vi "TestListen.vi"(0 "Input cluster":T1, 1 "Test Ready":bool, 2 "Loop Number":i32, 5 "Max No. of Tests":i32=3, 7 "Time to Complete":dbl, 9 "% Complete":i32, 11 "No. of Test":i32=1, 12 "TF IN":bool) -> (3 "Test No.":i32, 4 "Queue cluster":T1, 6 "Test Param":T2, 8 "Voltage/(g/s)":bool, 13 "TF OUT":bool, 14 "State":i32)   [LabVIEW 2014]
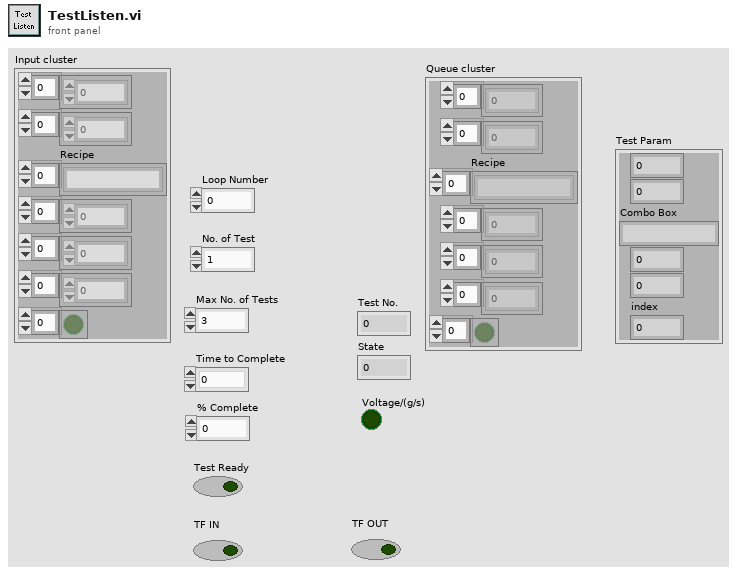
[diagram p1: front panel]
types:
  T1 = cluster{i32[], i32[], "Recipe":string[], i32[], i32[], i32[], bool[]}
  T2 = cluster{i32, i32, "Combo Box":string, i32, i32, "index":i32}
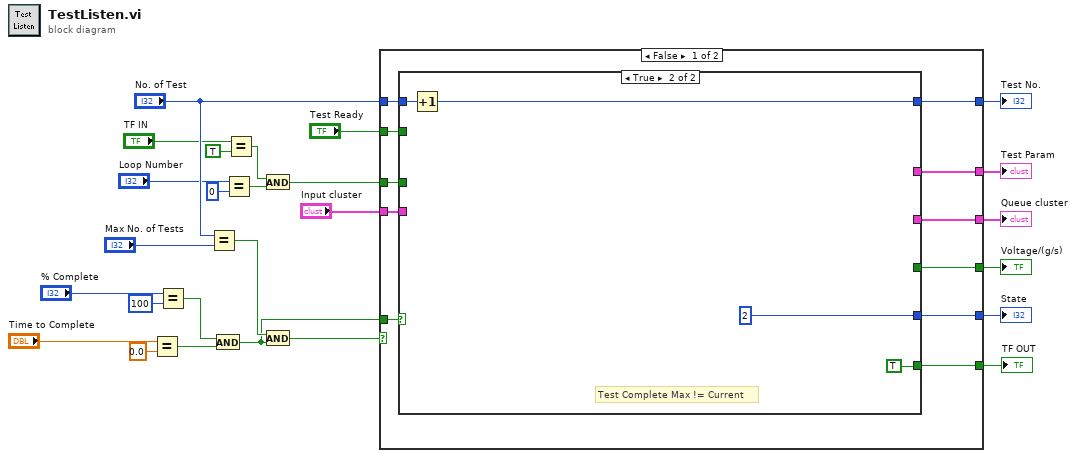
[diagram p0: block diagram]
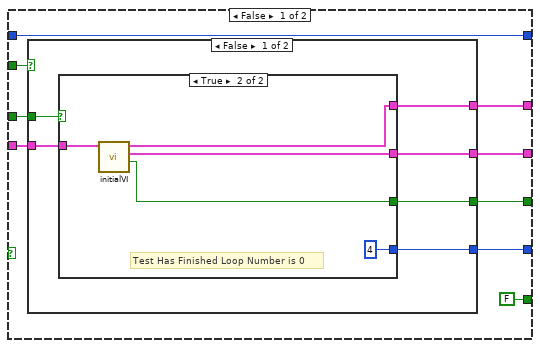
[diagram p2: hidden frame]
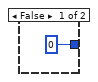
[diagram p3: hidden frame]
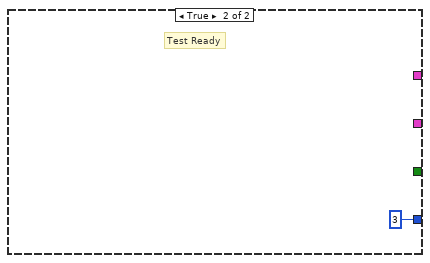
[diagram p4: hidden frame]
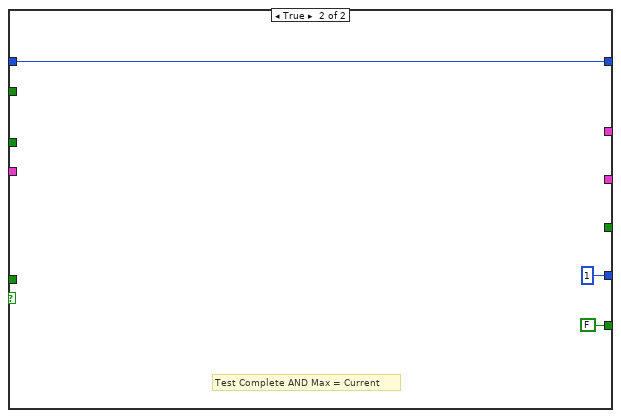
[diagram p5: hidden frame]
diagram:
  n1 = Equal?(x="Time to Complete", y=0.0) -> (x = y?=w24:bool)
  n2 = Equal?(x="% Complete", y=100) -> (x = y?=w25:bool)
  n3 = Equal?(x="No. of Test", y="Max No. of Tests") -> (x = y?=w26:bool)
  n4 = And(x=w25, y=w24) -> (x .and. y?=w21:bool)
  n5 = Equal?(x="Loop Number", y=0) -> (x = y?=w5:bool)
  n6 = Equal?(x="TF IN", y=TRUE) -> (x = y?=w3:bool)
  n7 = And(x=w3, y=w5) -> (x .and. y?=w2:bool)
  n8 = And(x=w26, y=w21) -> (x .and. y?=w22:bool)
  n9 = case shown="False" w22 {
    tunnel: w21 -> [w37 _]
    tunnel: "Test Ready" -> [w36 _]
    tunnel: [w35 1] -> w12
    tunnel: [w34 w65] -> w17
    tunnel: "No. of Test" -> [w33 w65]
    tunnel: w2 -> [w32 _]
    tunnel: "Input cluster" -> [w31 _]
    tunnel: [w30 _] -> w9
    tunnel: [w29 _] -> w11
    tunnel: [w28 _] -> w8
    tunnel: [w27 FALSE ("Test Ready 2")] -> w1
    frame False {
      n10 = case shown="True" w37 {
        tunnel: w36 -> [w45 _]
        tunnel: [w46 2] -> w35
        tunnel: [w44 w62] -> w34
        tunnel: w33 -> [w44 w61]
        tunnel: w32 -> [w43 _]
        tunnel: w31 -> [w42 _]
        tunnel: [w41 _] -> w30
        tunnel: [w40 _] -> w29
        tunnel: [w39 _] -> w28
        tunnel: [FALSE ("Test Ready 2") TRUE ("Test Ready 2")] -> w27
        frame False {
          n11 = case shown="False" w45 {
            tunnel: [w51 3] -> w46
            tunnel: w43 -> [w52 _]
            tunnel: w42 -> [w50 _]
            tunnel: [w49 _] -> w41
            tunnel: [w48 _] -> w40
            tunnel: [w47 _] -> w39
            frame False {
              n12 = case shown="True" w52 {
                tunnel: [0 4] -> w51
                tunnel: w50 -> [_ w55]
                tunnel: [_ w57] -> w49
                tunnel: [_ w56] -> w48
                tunnel: [_ w54] -> w47
                frame False {
                }
                frame True {
                  # "Test Has Finished Loop Number is 0"
                  n13 = call "initialVI.vi"("Input cluster"=w55) -> ("Voltage/(g/s)"=w54:bool, "Queue cluster"=w57:T1, "Test Param"=w56:T2)  [unwired: 7 in, 1 out]
                }
              }
            }
            frame True {
              # "Test Ready"
            }
          }
        }
        frame True {
          # "Test Complete Max != Current"
          n14 = Increment(x=w61) -> (x+1=w62:i32)
        }
      }
    }
    frame True {
      # "Test Complete AND Max = Current"
    }
  }
  "Test No." <- w17
  "State" <- w12
  "Test Param" <- w11
  "Queue cluster" <- w9
  "Voltage/(g/s)" <- w8
  "TF OUT" <- w1
